vi "Get ConfigFile Path.vi"(7 "create folder? (T)":bool=TRUE, 8 "error in (no error)":errorcluster, 11 "Artifactory in":refnum<class "Artifactory.lvclass">) -> (0 "error out":errorcluster, 1 "found":bool, 2 "Config File":path, 3 "Artifactory out":refnum<class "Artifactory.lvclass">)   [LabVIEW 2021, in "Artifactory.lvclass"]
uses:
  Artifactory.lvclass
  <vilib>/Utility/sysdir.llb/System Directory Type.ctl
  Artifactory.lvclass/Artifactory.ctl
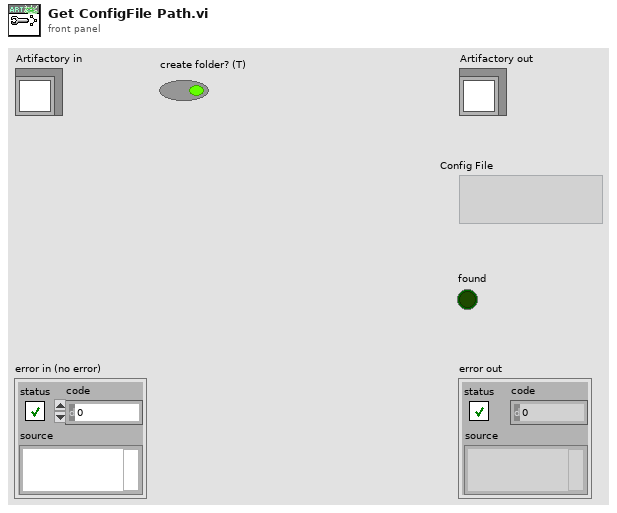
[diagram p1: front panel]
types:
  T1 = typedef "System Directory Type.ctl" = i32
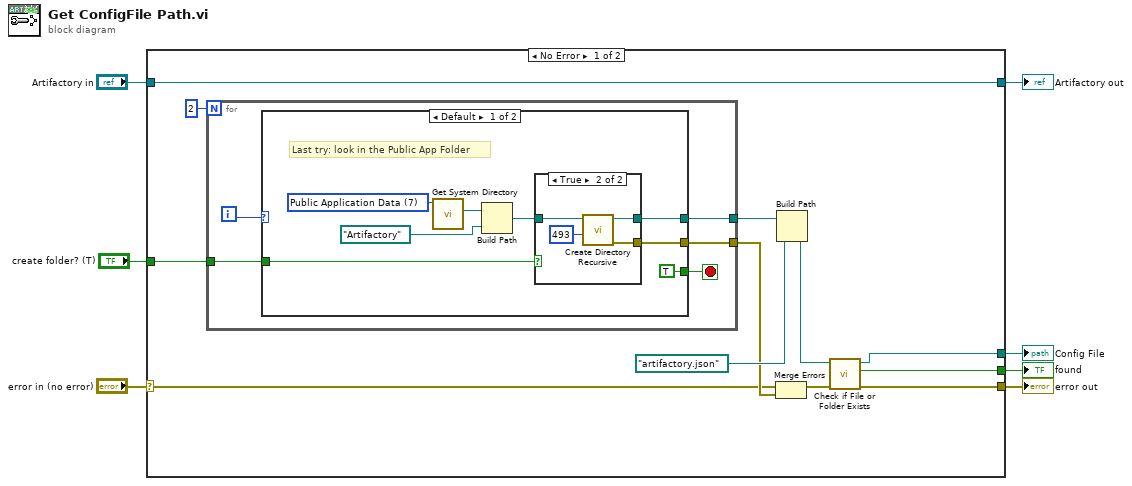
[diagram p0: block diagram]
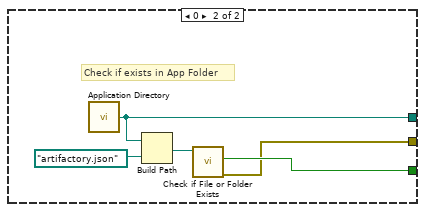
[diagram p3: hidden frame]
diagram:
  n1 = case shown="No Error" "error in (no error)" {
    selector: "error in (no error)" -> [w14 w44]
    tunnel: [w11 w44] -> w6
    tunnel: [w19 w43] -> w4
    tunnel: "Artifactory in" -> [w19 w43]
    tunnel: [w10 _] -> w3
    tunnel: "create folder? (T)" -> [w16 _]
    tunnel: [w13 _] -> w1
    frame No Error {
      n2 = for {
        N: 2 -> [_]
        tunnel: [w24] -> w17
        tunnel: w16 -> [w23]
        tunnel: [w22] -> w15
        i -> [w21]
        stop <- w20 stop-if-true
        n3 = case shown="Default" w21 {
          tunnel: [w28 w39] -> w24
          tunnel: w23 -> [w27 _]
          tunnel: [w26 w38] -> w22
          tunnel: [TRUE w40] -> w20
          frame Default {
            w32 = T1 7 items=["User Home"=0, "User Desktop"=1, "User Documents"=2, "User Application Data"=3, "User Preferences"=4, "User Temporary"=5, "Public Documents"=6, "Public Application Data"=7, "Public Preferences"=8, "Public Cache"=13, "System Core Libraries"=9, "System Installed Libraries"=10, "Application Files"=11, "Boot Volume Root"=12] ("system directory type")
            # "Last try: look in the Public App Folder"
            n4 = call <vilib>:"Get System Directory.vi"("system directory type"=w32) -> ("system directory"=w31:path)  [unwired: 10 in]
            n5 = Build Path(base path=w31, name or relative path=path "Artifactory") -> (appended path=w29:path)
            n6 = case shown="True" w27 {
              tunnel: w29 -> [w33 w37]
              tunnel: [w33 w36] -> w28
              tunnel: [_ w34] -> w26
              frame False {
              }
              frame True {
                n7 = call <vilib>:"Create Directory Recursive.vi"("permissions"=i16 493, "directory"=w37) -> ("error out"=w34:errorcluster, "directory copy"=w36:path)  [unwired: 3 in, 1 out]
              }
            }
          }
          frame 0 {
            # "Check if exists in App Folder"
            n8 = call <vilib>:"Application Directory.vi"() -> ("Application Directory"=w39:path)
            n9 = Build Path(base path=w39, name or relative path=path "artifactory.json") -> (appended path=w41:path)
            n10 = call <vilib>:"Check if File or Folder Exists.vi"("path"=w41) -> ("error out"=w38:errorcluster, "file or folder exists?"=w40:bool)  [unwired: 8 in, 1 out]
          }
        }
      }
      n11 = Merge Errors(w14, w15) -> (w12:errorcluster)
      n12 = Build Path(base path=w17, name or relative path=path "artifactory.json") -> (appended path=w9:path)
      n13 = call <vilib>:"Check if File or Folder Exists.vi"("error in (no error)"=w12, "path"=w9) -> ("error out"=w11:errorcluster, "file or folder exists?"=w13:bool, "dup path"=w10:path)  [unwired: 7 in]
    }
    frame Error {
    }
  }
  "error out" <- w6
  "Artifactory out" <- w4
  "Config File" <- w3
  "found" <- w1
